vi "Chaining Promises.vi"(8 "error in (no error)":errorcluster) -> (0 "error out":errorcluster)   [LabVIEW 2017, in "Unit Tests.lvlib"]
uses:
  Unit Tests.lvlib
  <vilib>/addons/_JKI Toolkits/Caraya/classes/Test/Test.lvclass
  <vilib>/addons/_JKI Toolkits/Caraya/classes/Assert/Assert.lvclass
  Promise/Promise/Promise.lvclass
  1ed7bcdd-aa0c-484d-85c7-5e62c30aac2b.vi
  3093b7d2-971d-487a-b662-131f608fd71a.vi
  f53b5818-9026-484c-88c8-97090a810389.vi
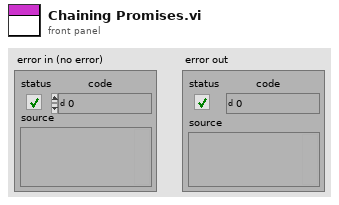
[diagram p1: front panel]
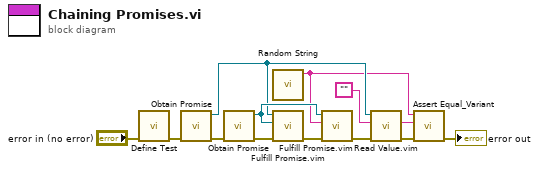
[diagram p0: block diagram]
diagram:
  n1 = call <vilib>:"Define Test.vi"("error in (no error)"="error in (no error)") -> ("error out"=w5:errorcluster)  [unwired: 10 in]
  n2 = call "Obtain Promise.vi"("error in (no error)"=w5) -> ("error out"=w10:errorcluster, "Promise out"=w9:refnum<class "Promise.lvclass">)  [unwired: 8 in, 1 out]
  n3 = call "Obtain Promise.vi"("error in (no error)"=w10) -> ("error out"=w11:errorcluster, "Promise out"=w13:refnum<class "Promise.lvclass">)  [unwired: 8 in, 1 out]
  n4 = call "Random String.vi"() -> ("string"=w2:string)  [unwired: 11 in]
  n5 = call "Fulfill Promise.vim"("error in (no error)"=w11, "Value"=w13, "Promise in"=w9) -> ("error out"=w12:errorcluster)  [unwired: 7 in, 1 out]
  n6 = call "Fulfill Promise.vim"("error in (no error)"=w12, "Value"=w2, "Promise in"=w13) -> ("error out"=w7:errorcluster)  [unwired: 7 in, 1 out]
  n7 = call "Read Value.vim"("error in (no error)"=w7, "Default Value"="", "Future in"=w9) -> ("error out"=w4:errorcluster, "Value"=w1:string)  [unwired: 5 in, 2 out]
  n8 = call <vilib>:"Assert Equal_Variant.vi"("error in (no error)"=w4, "Y"=w1, "X"=w2) -> ("error out"=→"error out":errorcluster)  [unwired: 8 in]
